vi "FUT_Save.vi"(0 "object in":refnum<class "SaveData.lvclass">, 2 "output cluster":T2, 3 "Oscilloscope Results 2":T1 {"Probe Current" format="%.2p"; "Phase Angle" format="%.2p"; "Main Freq" format="%.2p"; "Main Volt" format="%.2p"}, 4 "Temperature(C)":dbl, 5 "error in (no error)":errorcluster) -> (14 "object out":refnum<class "SaveData.lvclass">, 19 "error out":errorcluster)   [LabVIEW 2023, in "SaveData.lvclass"]
uses:
  SaveData.lvclass
  SaveData.lvclass/SaveData.ctl
  <vilib>/express/express shared/transition.llb/Dynamic To Waveform Array.vi
  <vilib>/express/express signal manip/GetorSetDDTAttributes/Set DDT Attributes/SetT0.vi
  <vilib>/express/express shared/transition.llb/Waveform Array To Dynamic.vi
  <vilib>/express/express signal manip/GetorSetDDTAttributes/Set DDT Attributes/Set DDT Properties.xnode
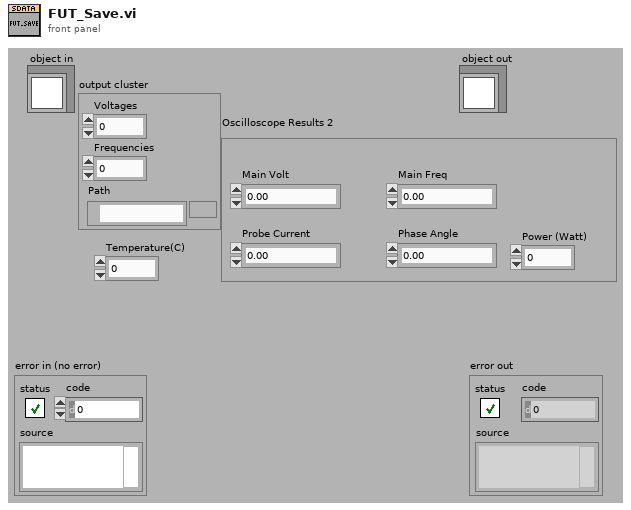
[diagram p1: front panel]
types:
  T1 = cluster{"Main Volt":dbl, "Main Freq":dbl, "Phase Angle":dbl, "Probe Current":dbl, "Power (Watt)":dbl}
  T2 = cluster{"Voltages":dbl, "Frequencies":dbl, "Path":path}
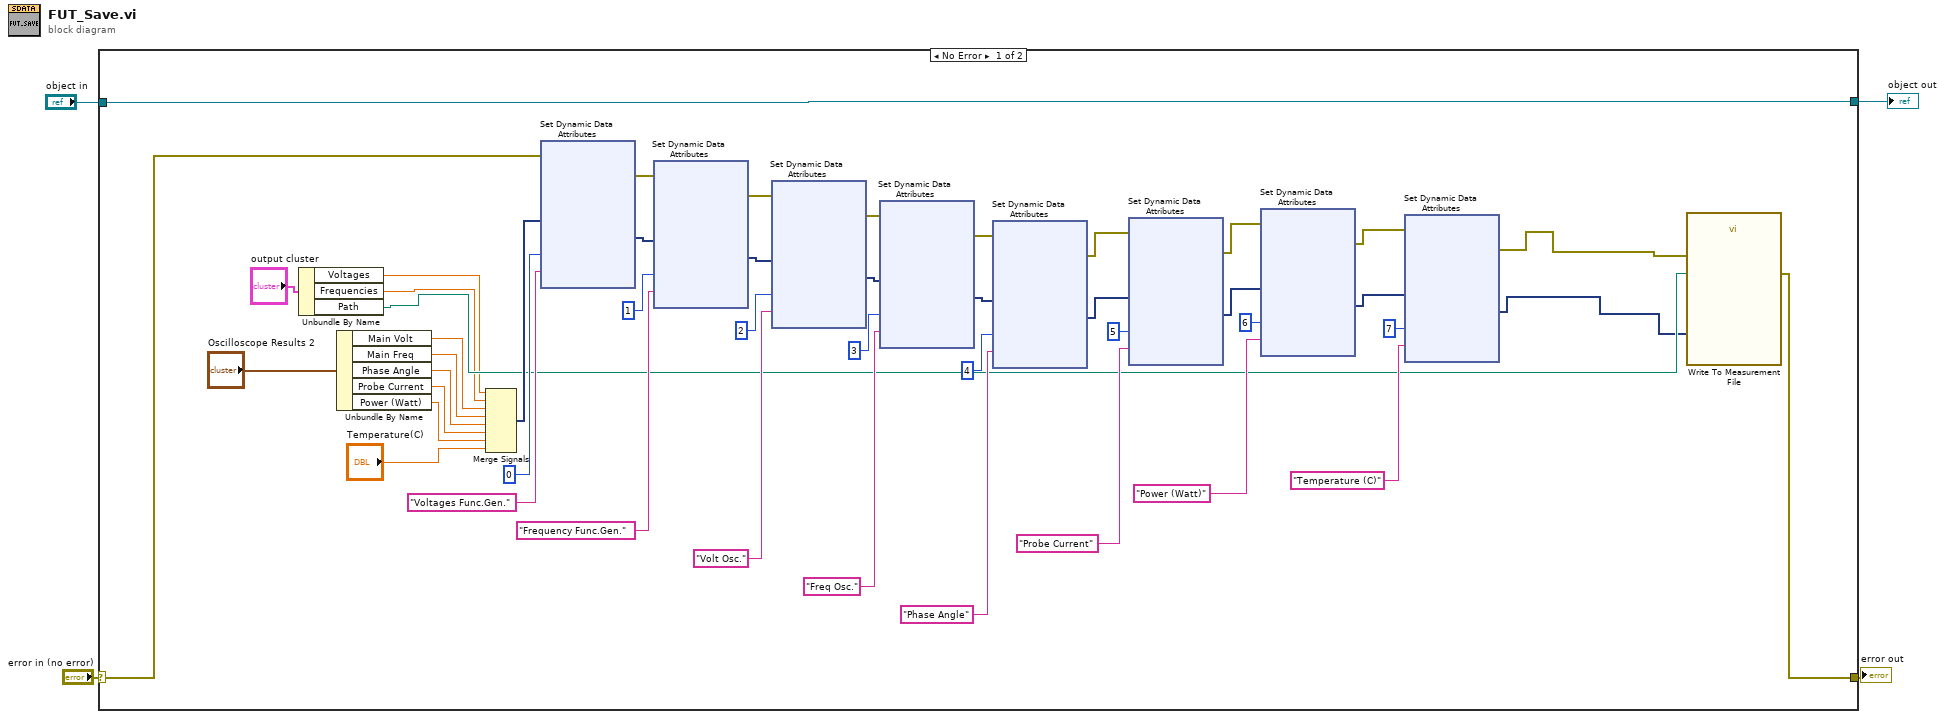
[diagram p0: block diagram]
diagram:
  n1 = case shown="No Error" "error in (no error)" {
    selector: "error in (no error)" -> [w10 w157]
    tunnel: [w9 w157] -> w3
    tunnel: [w51 w156] -> w1
    tunnel: "object in" -> [w51 w156]
    frame No Error {
      n2 = Unbundle By Name("output cluster") -> ("Voltages"=w6:dbl, "Frequencies"=w5:dbl, "Path"=w11:path)
      n3 = Unbundle By Name("Oscilloscope Results 2") -> ("Main Volt"=w36:dbl, "Main Freq"=w35:dbl, "Phase Angle"=w33:dbl, "Probe Current"=w27:dbl, "Power (Watt)"=w26:dbl)
      n4 = Merge Signals(w6, w5, w36, w35, w33, w27, w26, "Temperature(C)") -> (w34:dynamicdata)
      n5 = xnode "Set Dynamic Data Attributes"("Signals In"=w34, "Signal Index"=0, "Signal Name"="Voltages Func.Gen.", "error in"=w10) -> ("Signals Out"=w39:dynamicdata, "error out"=w48:errorcluster)
      n6 = xnode "Set Dynamic Data Attributes"("Signals In"=w39, "Signal Index"=1, "Signal Name"="Frequency Func.Gen.", "error in"=w48) -> ("Signals Out"=w38:dynamicdata, "error out"=w47:errorcluster)
      n7 = xnode "Set Dynamic Data Attributes"("Signals In"=w38, "Signal Index"=2, "Signal Name"="Volt Osc.", "error in"=w47) -> ("Signals Out"=w37:dynamicdata, "error out"=w46:errorcluster)
      n8 = xnode "Set Dynamic Data Attributes"("Signals In"=w37, "Signal Index"=3, "Signal Name"="Freq Osc.", "error in"=w46) -> ("Signals Out"=w31:dynamicdata, "error out"=w32:errorcluster)
      n9 = xnode "Set Dynamic Data Attributes"("Signals In"=w31, "Signal Index"=4, "Signal Name"="Phase Angle", "error in"=w32) -> ("Signals Out"=w21:dynamicdata, "error out"=w24:errorcluster)
      n10 = xnode "Set Dynamic Data Attributes"("Signals In"=w21, "Signal Index"=5, "Signal Name"="Probe Current", "error in"=w24) -> ("Signals Out"=w20:dynamicdata, "error out"=w23:errorcluster)
      n11 = xnode "Set Dynamic Data Attributes"("Signals In"=w20, "Signal Index"=6, "Signal Name"="Power (Watt)", "error in"=w23) -> ("Signals Out"=w19:dynamicdata, "error out"=w22:errorcluster)
      n12 = xnode "Set Dynamic Data Attributes"("Signals In"=w19, "Signal Index"=7, "Signal Name"="Temperature (C)", "error in"=w22) -> ("Signals Out"=w8:dynamicdata, "error out"=w7:errorcluster)
      n13 = call "Write To Measurement File"("Signals"=w8, "error in (no error)"=w7, "Filename"=w11) -> ("error out"=w9:errorcluster)  [unwired: 14 in, 2 out]
    }
    frame Error {
    }
  }
  "error out" <- w3
  "object out" <- w1
